vi "WritePhaseToCalcCache.vi"(6 "calc cache":variant, 9 "feature name":string, 10 "channel name":string, 11 "phase":dbl) -> (4 "calc cache out":variant)   [LabVIEW 2017, in "AnalysisHelper.lvlib"]
uses:
  <vilib>/addons/InsightCM/Utilities/Analysis/Shared/AnalysisHelper.lvlib
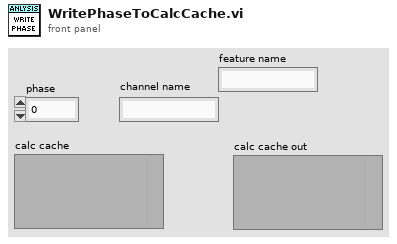
[diagram p1: front panel]
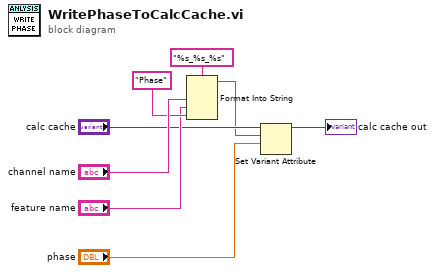
[diagram p0: block diagram]
diagram:
  n1 = Format Into String(format string="%s_%s_%s", "channel name", "feature name", "Phase" ("name")) -> (resulting string=w2:string)  [unwired: 2 in, 1 out]
  n2 = Set Variant Attribute(Variant="calc cache", name=w2, value="phase") -> (Variant out=→"calc cache out":variant)  [unwired: 1 in, 2 out]
